vi "PPL_PrivateClass_Test.vi"() -> ()   [LabVIEW 2017]
uses:
  <vilib>/addons/_JKI Toolkits/Caraya/classes/Assert/Assert Equal Value_Variant.vi
  <vilib>/addons/_JKI Toolkits/Caraya/classes/Assert/Assert Not Error.vi
  builds/TestLibrary/TestLibrary.lvlibp
  <vilib>/addons/_JKI Toolkits/Caraya/classes/Assert/Assert.lvclass
  <vilib>/addons/_JKI Toolkits/Caraya/classes/Test/Test.lvclass
panel:
  out "error out":errorcluster
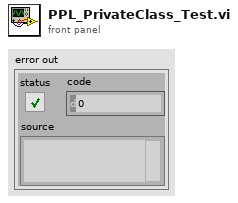
[diagram p1: front panel]
types:
  T1 = cluster{"Major":u16, "Minor":u16, "Fix":u16, "Build":u16}[]
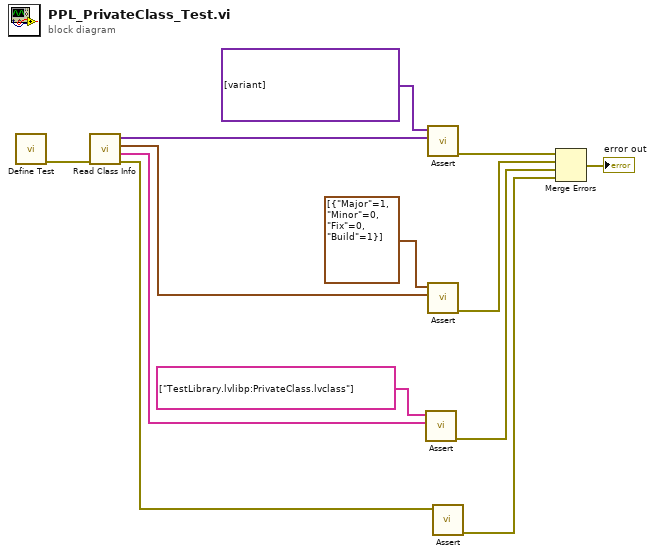
[diagram p0: block diagram]
diagram:
  n1 = call <vilib>:"Define Test.vi"() -> ("error out"=w1:errorcluster)  [unwired: 10 in, 1 out]
  n2 = call "Read Class Info.vi"("error in (no error)"=w1) -> ("error out"=w12:errorcluster, "Class Names"=w13:string[], "Library Versions"=w10:T1, "Private Data Clusters"=w8:variant[])  [unwired: 7 in]
  n3 = call-poly <vilib>:"Assert.vi"("Actual"=w13, "Expected"=string[] ["TestLibrary.lvlibp:PrivateClass.lvclass"] ("Class Names")) -> ("error out"=w4:errorcluster)  [unwired: 8 in, 1 out]
  n4 = call-poly <vilib>:"Assert.vi"("Actual"=w8, "Expected"=variant[] [variant(cluster{"String":string} {"String"="Hello World!"})] ("Private Data Clusters")) -> ("error out"=w6:errorcluster)  [unwired: 8 in, 1 out]
  n5 = call-poly <vilib>:"Assert.vi"("Actual"=w10, "Expected"=T1 [{"Major"=1, "Minor"=0, "Fix"=0, "Build"=1}] ("Library Versions")) -> ("error out"=w5:errorcluster)  [unwired: 8 in, 1 out]
  n6 = call-poly <vilib>:"Assert.vi"("Not Error?"=w12) -> ("error out"=w3:errorcluster)  [unwired: 9 in, 1 out]
  n7 = Merge Errors(w6, w5, w4, w3) -> (→"error out":errorcluster)
